vi "Linux Scan DNS Config.vi"(8 "error in (no error)":errorcluster) -> (0 "error out":errorcluster, 3 "DNS server addresses":refnum<class "Generic Network Address.lvclass">[](array[class]))   [LabVIEW 2020, in "NI_WFCN.lvlib" / "Hostname Network Address.lvclass"]
doc: "Linux: Attempt to locate configured DNS servers."
uses:
  <vilib>/net/WFCN/Addressing/Hostname Network Address/Hostname Network Address.lvclass
  <vilib>/net/WFCN/Addressing/Generic Network Address/Generic Network Address.lvclass
  <vilib>/net/WFCN/Addressing/IPv4 Network Address/IPv4 Network Address.lvclass
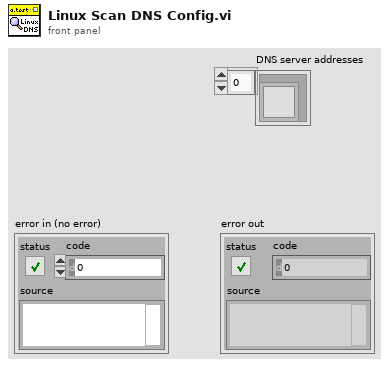
[diagram p1: front panel]
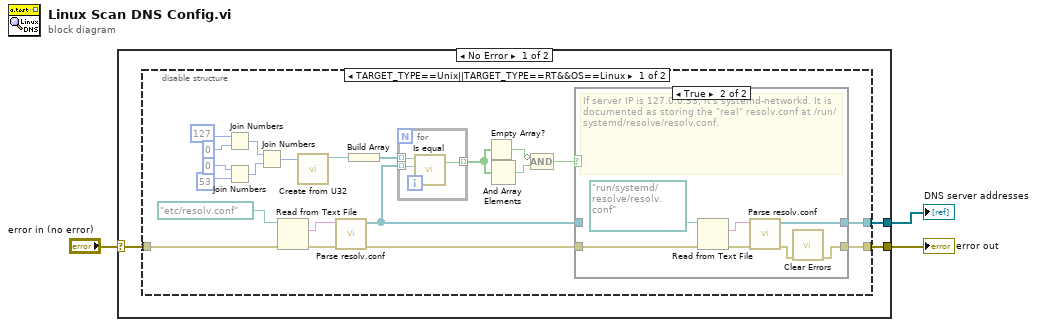
[diagram p0: block diagram]
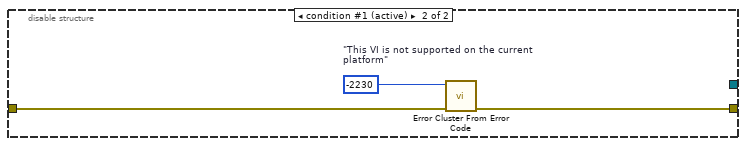
[diagram p3: hidden frame]
diagram:
  n1 = case shown="No Error" "error in (no error)" {
    selector: "error in (no error)" -> [w4 w43]
    tunnel: [w6 w43] -> w3
    tunnel: [w5 _] -> w2
    frame No Error {
      n2 = disable-structure shown="TARGET_TYPE==Unix||TARGET_TYPE==RT&&OS==Linux" {
        disable-tunnel: w4 -> [w26 w41]
        disable-tunnel: [w14 w40] -> w6
        disable-tunnel: [w11 _] -> w5
        frame condition #0 {
          n3 = Join Numbers(hi=u8 127, lo=u8 0) -> ((hi.lo)=w18:u16)
          n4 = Join Numbers(hi=u8 0, lo=u8 53) -> ((hi.lo)=w19:u16)
          n5 = Join Numbers(hi=w18, lo=w19) -> ((hi.lo)=w17:u32)
          n6 = Read from Text File(file (use dialog)=path "/etc/resolv.conf", error in=w26) -> (text=w24:string, error out=w25:errorcluster)  [unwired: 2 in, 2 out]
          n7 = call <vilib>:"Create from U32.vi"("address U32"=w17) -> ("address out"=w13:refnum<class "IPv4 Network Address.lvclass">)  [unwired: 10 in]
          n8 = call <vilib>:"Parse resolv.conf.vi"("error in (no error)"=w25, "resolv.conf contents"=w24) -> ("error out"=w16:errorcluster, "DNS server addresses"=w15:refnum<class "Generic Network Address.lvclass">[])  [unwired: 8 in]
          n9 = Build Array(w13) -> (w12:refnum<class "IPv4 Network Address.lvclass">[])
          n10 = for {
            tunnel: [w28] -> w10 mode=indexing
            tunnel: w15 -> [w29] mode=indexing
            tunnel: w12 -> [w30] mode=indexing
            n11 = call-dynamic "Is equal.vi"("address 2"=w29, "address"=w30) -> ("equal?"=w28:bool)  [unwired: 3 in]
          }
          n12 = Empty Array?(array=w10) -> (empty?=w8:bool)
          n13 = And Array Elements(Boolean array=w10) -> (logical AND=w9:bool)
          n14 = Compound Arithmetic op=AND(invert w8, w9) -> (w7:bool)
          n15 = case shown="True" w7 {
            tunnel: w16 -> [w31 w38]
            tunnel: [w32 w35] -> w11
            tunnel: [w31 w33] -> w14
            tunnel: w15 -> [w32 _]
            frame False {
              # "If it's otherwise 127.*, it's a caching nameserver, but we don't know where the real config is, so just assume it's ok.\n\nOtherwise if we got a nameserver then assume it's configured and exit."
            }
            frame True {
              # "If server IP is 127.0.0.53, it's systemd-networkd. It is documented as storing the \"real\" resolv.conf at /run/systemd/resolve/resolv.conf."
              n16 = Read from Text File(file (use dialog)=path "/run/systemd/resolve/resolv.conf", error in=w38) -> (text=w36:string, error out=w37:errorcluster)  [unwired: 2 in, 2 out]
              n17 = call <vilib>:"Parse resolv.conf.vi"("error in (no error)"=w37, "resolv.conf contents"=w36) -> ("error out"=w34:errorcluster, "DNS server addresses"=w35:refnum<class "Generic Network Address.lvclass">[])  [unwired: 8 in]
              n18 = call <vilib>:"Clear Errors.vi"("error in (no error)"=w34) -> ("error out"=w33:errorcluster)  [unwired: 5 in, 1 out]
            }
          }
        }
        frame condition #1 (active) {
          w42 = -2230  # "This VI is not supported on the current platform"
          n19 = call <vilib>:"Error Cluster From Error Code.vi"("error in (no error)"=w41, "error code (0)"=w42) -> ("error out"=w40:errorcluster)  [unwired: 7 in]
        }
      }
    }
    frame Error {
    }
  }
  "error out" <- w3
  "DNS server addresses" <- w2
